vi "Diagram Node Information.vi"(7 "InnerTerminal in":refnum<vi>[](array[refnum]), 8 "error in (no error)":errorcluster, 10 "Array in":refnum<vi>[](array[refnum]), 11 "Front Tunnels":refnum<vi>[](array[refnum])) -> (0 "error out":errorcluster, 1 "Array":cluster{i32, "ClassName":string}[](array[cluster]), 3 "Array out":T1[](array[typedef]))   [LabVIEW 2017, in "CSM-Helper.lvclass"]
doc: "### Diagram Node Information.vi\n\n-- <b>Controls</b> --\n- <b>InnerTerminal in</b>:\n- <b>Array in</b>:\n- <b>Front Tunnels</b>:\n\n-- <b>Indicators</b> --\n- <b>Array</b>:\n- <b>Array out</b>:"
uses:
  CSM-Helper.lvclass
  Utility/_Support/Diagram.llb/Def-Conncted Information.ctl
  <vilib>/Utility/miscctls.llb/LVPositionTypeDef.ctl
  Utility/_Support/Terminals.llb/csmHelper-Terminals.lvlib
  Utility/_Support/Diagram.llb/csmHelper-Diagram.lvlib
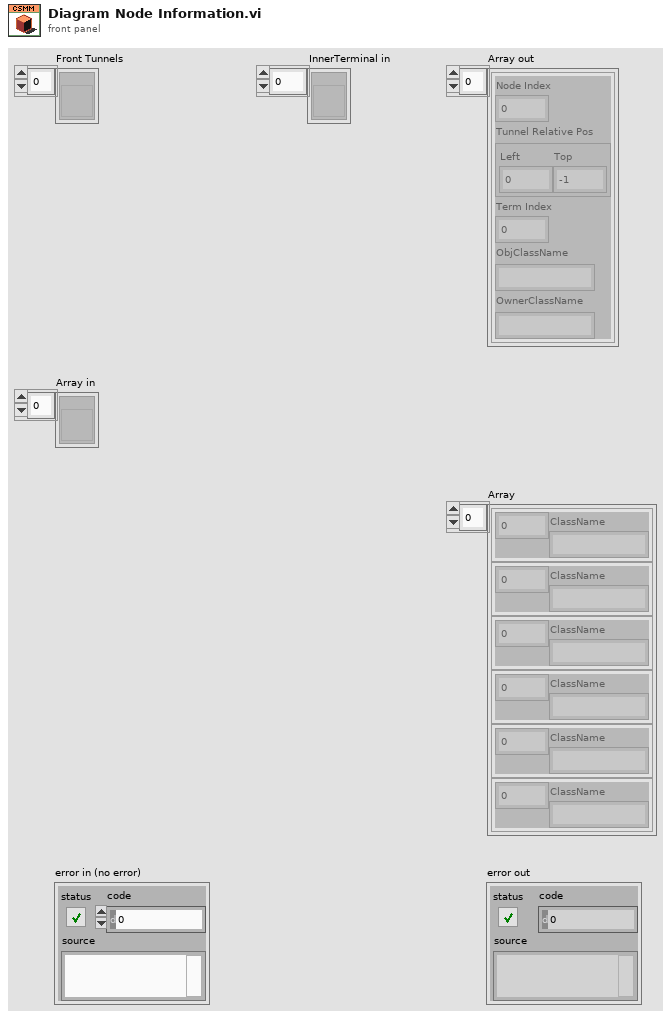
[diagram p1: front panel]
types:
  T1 = typedef "csmHelper-Diagram.lvlib/Def-Conncted Information.ctl" = cluster{"Node Index":i32, "Tunnel Relative Pos":T2, "Term Index":i32, "ObjClassName":string, "OwnerClassName":string}
  T2 = typedef "LVPositionTypeDef.ctl" = cluster{"Left":i32, "Top":i32}
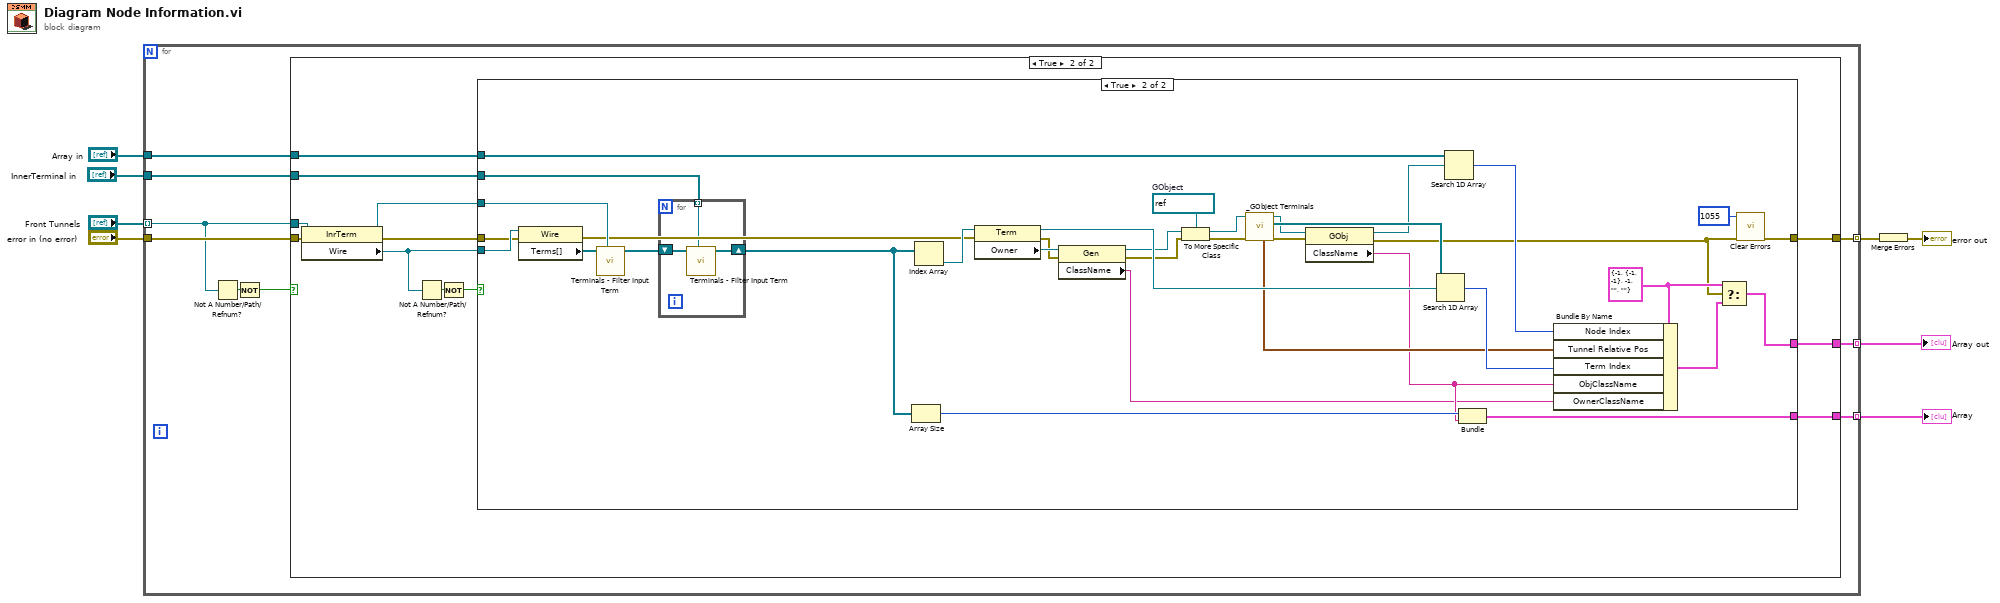
[diagram p0: block diagram]
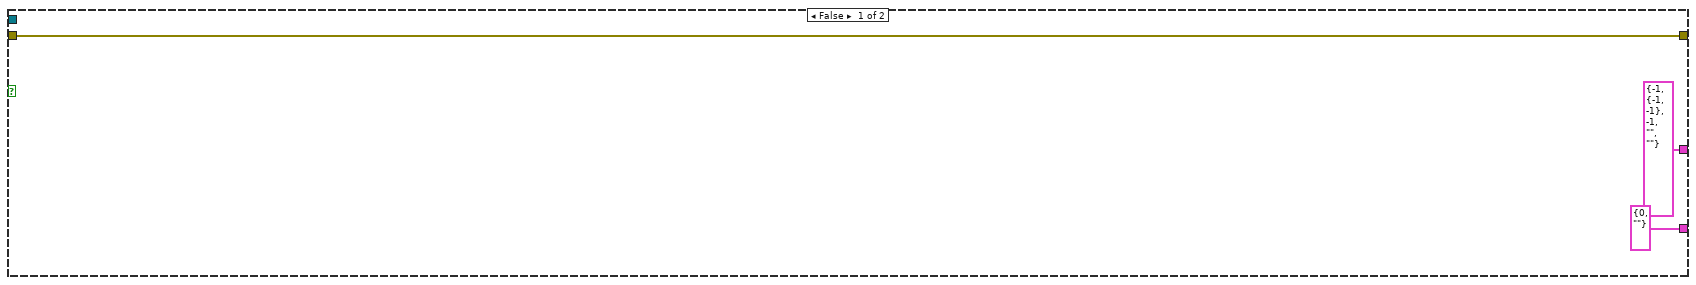
[diagram p2: hidden frame]
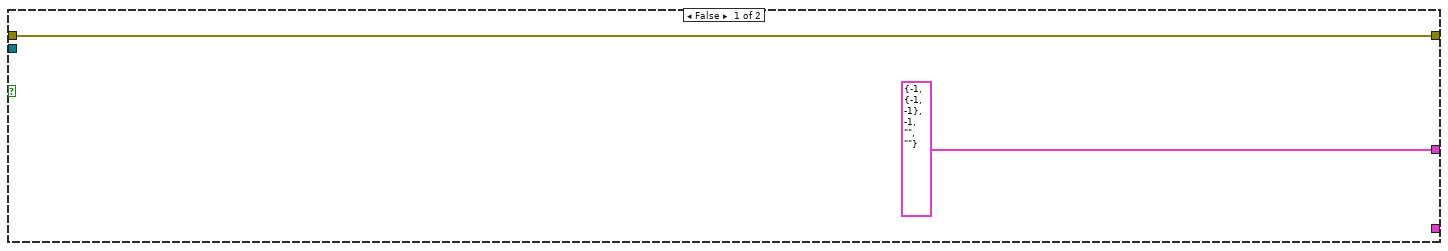
[diagram p3: hidden frame]
diagram:
  n1 = for {
    tunnel: "Array in" -> [w17]
    tunnel: [w14] -> w6 mode=indexing
    tunnel: "Front Tunnels" -> [w10] mode=indexing
    tunnel: "error in (no error)" -> [w16]
    tunnel: [w15] -> w3 mode=indexing
    tunnel: [w13] -> w2 mode=indexing
    tunnel: "InnerTerminal in" -> [w12]
    n2 = Not A Number/Path/Refnum?(number/path/refnum=w10) -> (NaN/Path/Refnum?=w11:bool)
    n3 = Not(x=w11) -> (.not. x?=w9:bool)
    n4 = case shown="True" w9 {
      tunnel: w17 -> [_ w32]
      tunnel: w16 -> [w20 w31]
      tunnel: [w20 w28] -> w15
      tunnel: [T1 {"Node Index"=-1, "Tunnel Relative Pos"={"Left"=-1, "Top"=-1}, "Term Index"=-1, "ObjClassName"="", "OwnerClassName"=""} ("cluster") w27] -> w14
      tunnel: [cluster{i32, "ClassName":string} {0, "ClassName"=""} w24] -> w13
      tunnel: w12 -> [_ w23]
      tunnel: w10 -> [_ w21]
      frame False {
      }
      frame True {
        n5 = property class="InrTerm"(reference=w21, error in=w31) -> (reference out=w29:refnum<vi>, error out=w30:errorcluster, "Wire"=w25:refnum<vi>)
        n6 = Not A Number/Path/Refnum?(number/path/refnum=w25) -> (NaN/Path/Refnum?=w26:bool)
        n7 = Not(x=w26) -> (.not. x?=w22:bool)
        n8 = case shown="True" w22 {
          tunnel: w32 -> [_ w59]
          tunnel: w25 -> [_ w69]
          tunnel: w30 -> [w34 w68]
          tunnel: w29 -> [_ w66]
          tunnel: [w34 w62] -> w28
          tunnel: [T1 {"Node Index"=-1, "Tunnel Relative Pos"={"Left"=-1, "Top"=-1}, "Term Index"=-1, "ObjClassName"="", "OwnerClassName"=""} ("cluster") w60] -> w27
          tunnel: [_ w55] -> w24
          tunnel: w23 -> [_ w37]
          frame False {
          }
          frame True {
            w51 = T1 {"Node Index"=-1, "Tunnel Relative Pos"={"Left"=-1, "Top"=-1}, "Term Index"=-1, "ObjClassName"="", "OwnerClassName"=""} ("cluster")
            w58 = refnum<vi> refnum  # GObject
            n9 = property class="Wire"(reference=w69, error in=w68) -> (error out=w64:errorcluster, "Terms[]"=w67:refnum<vi>[])  [unwired: 1 out]
            n10 = call "Terminals - Filter Input Term.vi"("InnerTerminal in"=w66, "Wire.Terms[] in"=w67) -> ("Wire.Terms[] out"=w39:refnum<vi>[])  [unwired: 9 in]
            n11 = for {
              shift-right: [w71] -> w38
              shift-left: w39 -> [w72]
              tunnel: w37 -> [w70] mode=indexing
              n12 = call "Terminals - Filter Input Term.vi"("InnerTerminal in"=w70, "Wire.Terms[] in"=w72) -> ("Wire.Terms[] out"=w71:refnum<vi>[])  [unwired: 9 in]
            }
            n13 = Array Size(array=w38) -> (size(s)=w56:i32)
            n14 = Index Array(array=w38) -> (element=w65:refnum<vi>)  [unwired: 1 in]
            n15 = property class="Term"(reference=w65, error in=w64) -> (reference out=w63:refnum<vi>, error out=w42:errorcluster, "Owner"=w44:refnum<vi>)
            n16 = property class="Gen"(reference=w44, error in=w42) -> (reference out=w43:refnum<vi>, error out=w41:errorcluster, "ClassName"=w40:string)
            n17 = To More Specific Class(target class=w58, reference=w43, error in=w41) -> (specific class reference=w53:refnum<vi>, error out=w54:errorcluster)
            n18 = call "_GObject Terminals.vi"("error in (no error)"=w54, "GObject in"=w53) -> ("error in (no error) (dup)"=w36:errorcluster, "Terms[]"=w52:refnum<vi>[], "Node Object"=w47:refnum<vi>, "tunnel Relative Pos"=w48:T2)  [unwired: 5 in, 1 out]
            n19 = property class="GObj"(reference=w47, error in=w36) -> (reference out=w46:refnum<vi>, error out=w35:errorcluster, "ClassName"=w45:string)
            n20 = Search 1D Array(1D array=w52, element=w63) -> (index of element=w49:i32)  [unwired: 1 in]
            n21 = Search 1D Array(1D array=w59, element=w46) -> (index of element=w57:i32)  [unwired: 1 in]
            n22 = Bundle(w56, "ClassName"=w45) -> (w55:cluster{i32, "ClassName":string})  [unwired: 1 in]
            n23 = Bundle By Name(cluster=w51, "Node Index"=w57, "Tunnel Relative Pos"=w48, "Term Index"=w49, "ObjClassName"=w45, "OwnerClassName"=w40) -> (w50:T1)
            n24 = Select(t=w51, s=w35, f=w50) -> (s? t:f=w60:T1)
            n25 = call <vilib>:"Clear Errors.vi"("error in (no error)"=w35, "specific error code to clear (0: all)"=1055) -> ("error out"=w62:errorcluster)  [unwired: 4 in, 1 out]
          }
        }
      }
    }
  }
  "Array out" <- w6
  "Array" <- w2
  n26 = Merge Errors(w3) -> (→"error out":errorcluster)
